vi "PID_Trajectory tracking_0125.vi"() -> ()   [LabVIEW 2018]
doc: "Demonstrates the use of the Network Streams functions to send LED status to the myRIO target."
uses:
  <vilib>/ErrorRing/Error Ring.xnode
  <vilib>/vision/NI_Vision_Development_Module.lvlib
panel:
  out "e(t-1)":dbl[](array[numeric])
  out "Ki part":dbl[](array[numeric])
  out "Kd part":dbl[](array[numeric])
  out "Kp part":dbl[](array[numeric])
  out "desired_relative_end_point_y":dbl
  out "desired_relative_end_point_x":dbl
  out "predicted_output_pr":dbl
  out "predicted_output_dr":dbl
  out "u(t)":dbl[](array[numeric])
  in  "Ki: Intergrate":dbl
  in  "Kd: Derivative":dbl[](array[numeric])
  in  "T":dbl[](array[numeric])
  in  "Kp: Proportional":dbl[](array[numeric])
  out "error  e(t)":dbl[](array[numeric])
  out "error_end_point_y":dbl
  out "error_end_point_x":dbl
  out "relative_end_point_y":dbl
  out "relative_end_point_x":dbl
  out "magnet_input_pr":dbl
  out "magnet_input_dr":dbl
  in  "打开仅尖端轨迹":bool
  out "仅尖端轨迹":T1(plugin-control)
  out "Bounding Box.Y Top":i32
  out "Bounding Box.X Left":i32
  out "curve_min_y":dbl
  out "curve_min_x":dbl
  out "curve_max_y":dbl
  out "curve_max_x":dbl
  out "relative_end_point_y":dbl
  out "relative_end_point_x":dbl
  out "delta_y":dbl
  out "delta_x":dbl
  out "pr":dbl
  out "tan(v)":dbl
  out "delta_velocity":dbl format="%#_10g"
  out "delta_time":dbl
  out "now time":timestamp[](array[timestamp])
  out "prev time":timestamp[](array[timestamp])
  out "delta_distance":dbl
  out "prev_end_point_y":dbl
  out "prev_end_point_x":dbl
  out "now_end_point_y":dbl
  out "now_end_point_x":dbl
  out "prev_end_point_y":dbl[](array[numeric])
  out "prev_end_point_x":dbl[](array[numeric])
  out "dr":dbl
  in  "Ar":sgl=11.0
  out "all parameters":dbl[][](array[numeric])
  out "direction angle":sgl[](array[numeric])
  out "dr":sgl
  out "strength":dbl[](array[numeric])
  out "场强":dbl
  out "end_point_y":T2
  out "end_point_x":dbl[](array[numeric])
  out "start_point_y":dbl[](array[numeric])
  out "start_point_x":dbl[](array[numeric])
  out "T":i32[](array[numeric])
  out "c":dbl[](array[numeric])
  out "b":dbl[](array[numeric])
  out "a\na":dbl[](array[numeric])
  out "c":dbl
  out "b":dbl
  out "a":dbl
  out "Angles (deg)":sgl[](array[numeric]) format="%.2f"
  in  "wr":sgl
  in  "打开轨迹":bool
  out "中心轨迹和尖端轨迹":T1(plugin-control)
  out "end_y":dbl
  out "end_x":dbl
  out "start_y":dbl
  out "start_x":dbl
  out "Image Pixels (U8)":u8[][](array[numeric])
  in  "Poly":dbl
  out "中心轨迹":T1(plugin-control)
  in  "保存按钮":bool
  out "Object Center":cluster{"X":sgl, "Y":sgl}
  out "黑白图":T1(plugin-control)
  in  "Number of Erosion":i32=5
  in  "Settings":T3={"Objects"=1, "Threshold"=128, "Reject Border"=FALSE, "Fill Holes"=FALSE, "Min Object Size"=TRUE, "Min Size"=5500, "Max Object Size"=FALSE, "Max Size"=100, "Show Search Area"=TRUE, "Show Center"=TRUE, "Show Bounding Box"=TRUE} {"Objects" items=["Bright Objects", "Dark Objects"]; "Threshold" min=1 max=999999999 step=1; "Max Size" min=1 max=999999999 step=1; "Min Size" min=1 max=999999999 step=1}
  out "Objects":T4(array[cluster]) {"Aspect Ratio" format="%.2f"; "Orientation" format="%.2f"; "Area" format="%.2f"; "Object Center"."Y" format="%.2f"; "Object Center"."X" format="%.2f"}
  in  "Search Rect (entire image)":T5={"Left"=160, "Top"=740, "Right"=1900, "Bottom"=1620, "Rotation"=0.0} {"Rotation" format="%.2f"; "Left" scale=0.0..1024.0; "Right" scale=0.0..1024.0}
  in  "Range":cluster{"Lower value":sgl, "Upper value":sgl}={"Lower value"=170.0, "Upper value"=255.0} {"Upper value" format="%.2f"; "Lower value" format="%.2f"}
  out "原图":T1(plugin-control)
  in  "停止":bool
  out "T":i32
  out "T":i32
  in  "磁场变换":bool=TRUE
  in  "Pause":bool
  out "Array":dbl[](array[numeric])
  in  "Parameter Settings":T6(tab)=enum."Rotating Field" caption="Field Types"
  in  "Ag":dbl
  in  "dg":dbl
  in  "pg":dbl
  in  "fg":dbl
  in  "AoOF":dbl
  in  "fo":sgl
  in  "do":sgl
  in  "oo":sgl
  in  "po":sgl
  in  "cc":sgl
  in  "pc":sgl
  in  "wc":sgl
  in  "dc":sgl
  in  "Ac":dbl
  in  "Dis phase step":dbl
  in  "Dis phase frequency (Hz)":dbl
  in  "Dis tumbling frequency (Hz)":dbl
  in  "Dis strength(mT)":dbl
  in  "Swa strength (mT)":dbl
  in  "Swa frequency (Hz)":dbl
  in  "Swa pitch angle (deg)":dbl
  in  "Swa direction angle (deg)":dbl
  in  "Swa ratio":dbl=1.0
  in  "Pitch Angle (rotating around Constant, deg)":dbl
  in  "Ratio (A/C)":sgl
  in  "Direction Angle (deg)":sgl
  in  "Pitch Angle (rotating around Origin, deg)":sgl
  in  "Frequency (Hz)":sgl
  in  "Strength (mT)":dbl
  in  "Ar 2":dbl caption="Ar"
  in  "ratio":sgl
  in  "pr  2":sgl
  in  "dr  2":sgl
  in  "wr  2":sgl
  in  "p_x":sgl
  out "Numeric 5":i32
  in  "Stop":bool
  out "error out":errorcluster
  in  "Target IP Address":string="172.22.11.2"
  # "Overview: Magnetic field calculation, and send parameters to myRIO\nInstructions:\n1. Verify the value of Target IP Address. Set Visa resource name.\n2. Ensure RT Main.vi is already running. \n3. Run this VI. Set parameters of magnetic field."
  # "Strength (mT)"
  # "Frequency (Hz)"
  # "Pitch Angle (deg)"
  # "Direction Angle (deg)"
  # "Strength (mT)"
  # "Pitch Angle (deg)"
  # "Direction Angle (deg)"
  # "Frequency (Hz)"
  # "Strength (mT)"
  # "Oscilation Frequency (Hz)"
  # "Oscilation Angle (deg)"
  # "Pitch Angle (deg)"
  # "Direction Angle (deg)"
  # "Strength (mT)"
  # "Frequency (Hz)"
  # "Pitch Angle (deg)"
  # "Direction Angle (deg)"
  # "Conical Angle (deg)"
  # "Strength (mT)"
  # "Tumbling Frequency (Hz)"
  # "Phase Frequency (Hz)"
  # "Phase Step"
  # "Strength (mT)"
  # "Frequency (Hz)"
  # "Pitch Angle (deg)"
  # "Direction Angle (deg)"
  # "Ratio"
  # "Strength (mT)"
  # "Frequency (Hz)"
  # "Ratio (A/C)"
  # "Direction Angle (deg)"
  # "Pitch Angle (rotating around Origin, deg)"
  # "Pitch Angle (rotating around Constant, deg)"
  # "Strength (mT)"
  # "Frequency (Hz)"
  # "Pitch Angle Y (deg)"
  # "Pitch Angle X (deg)"
  # "Direction Angle (deg)"
  # "ratio (l/s)"
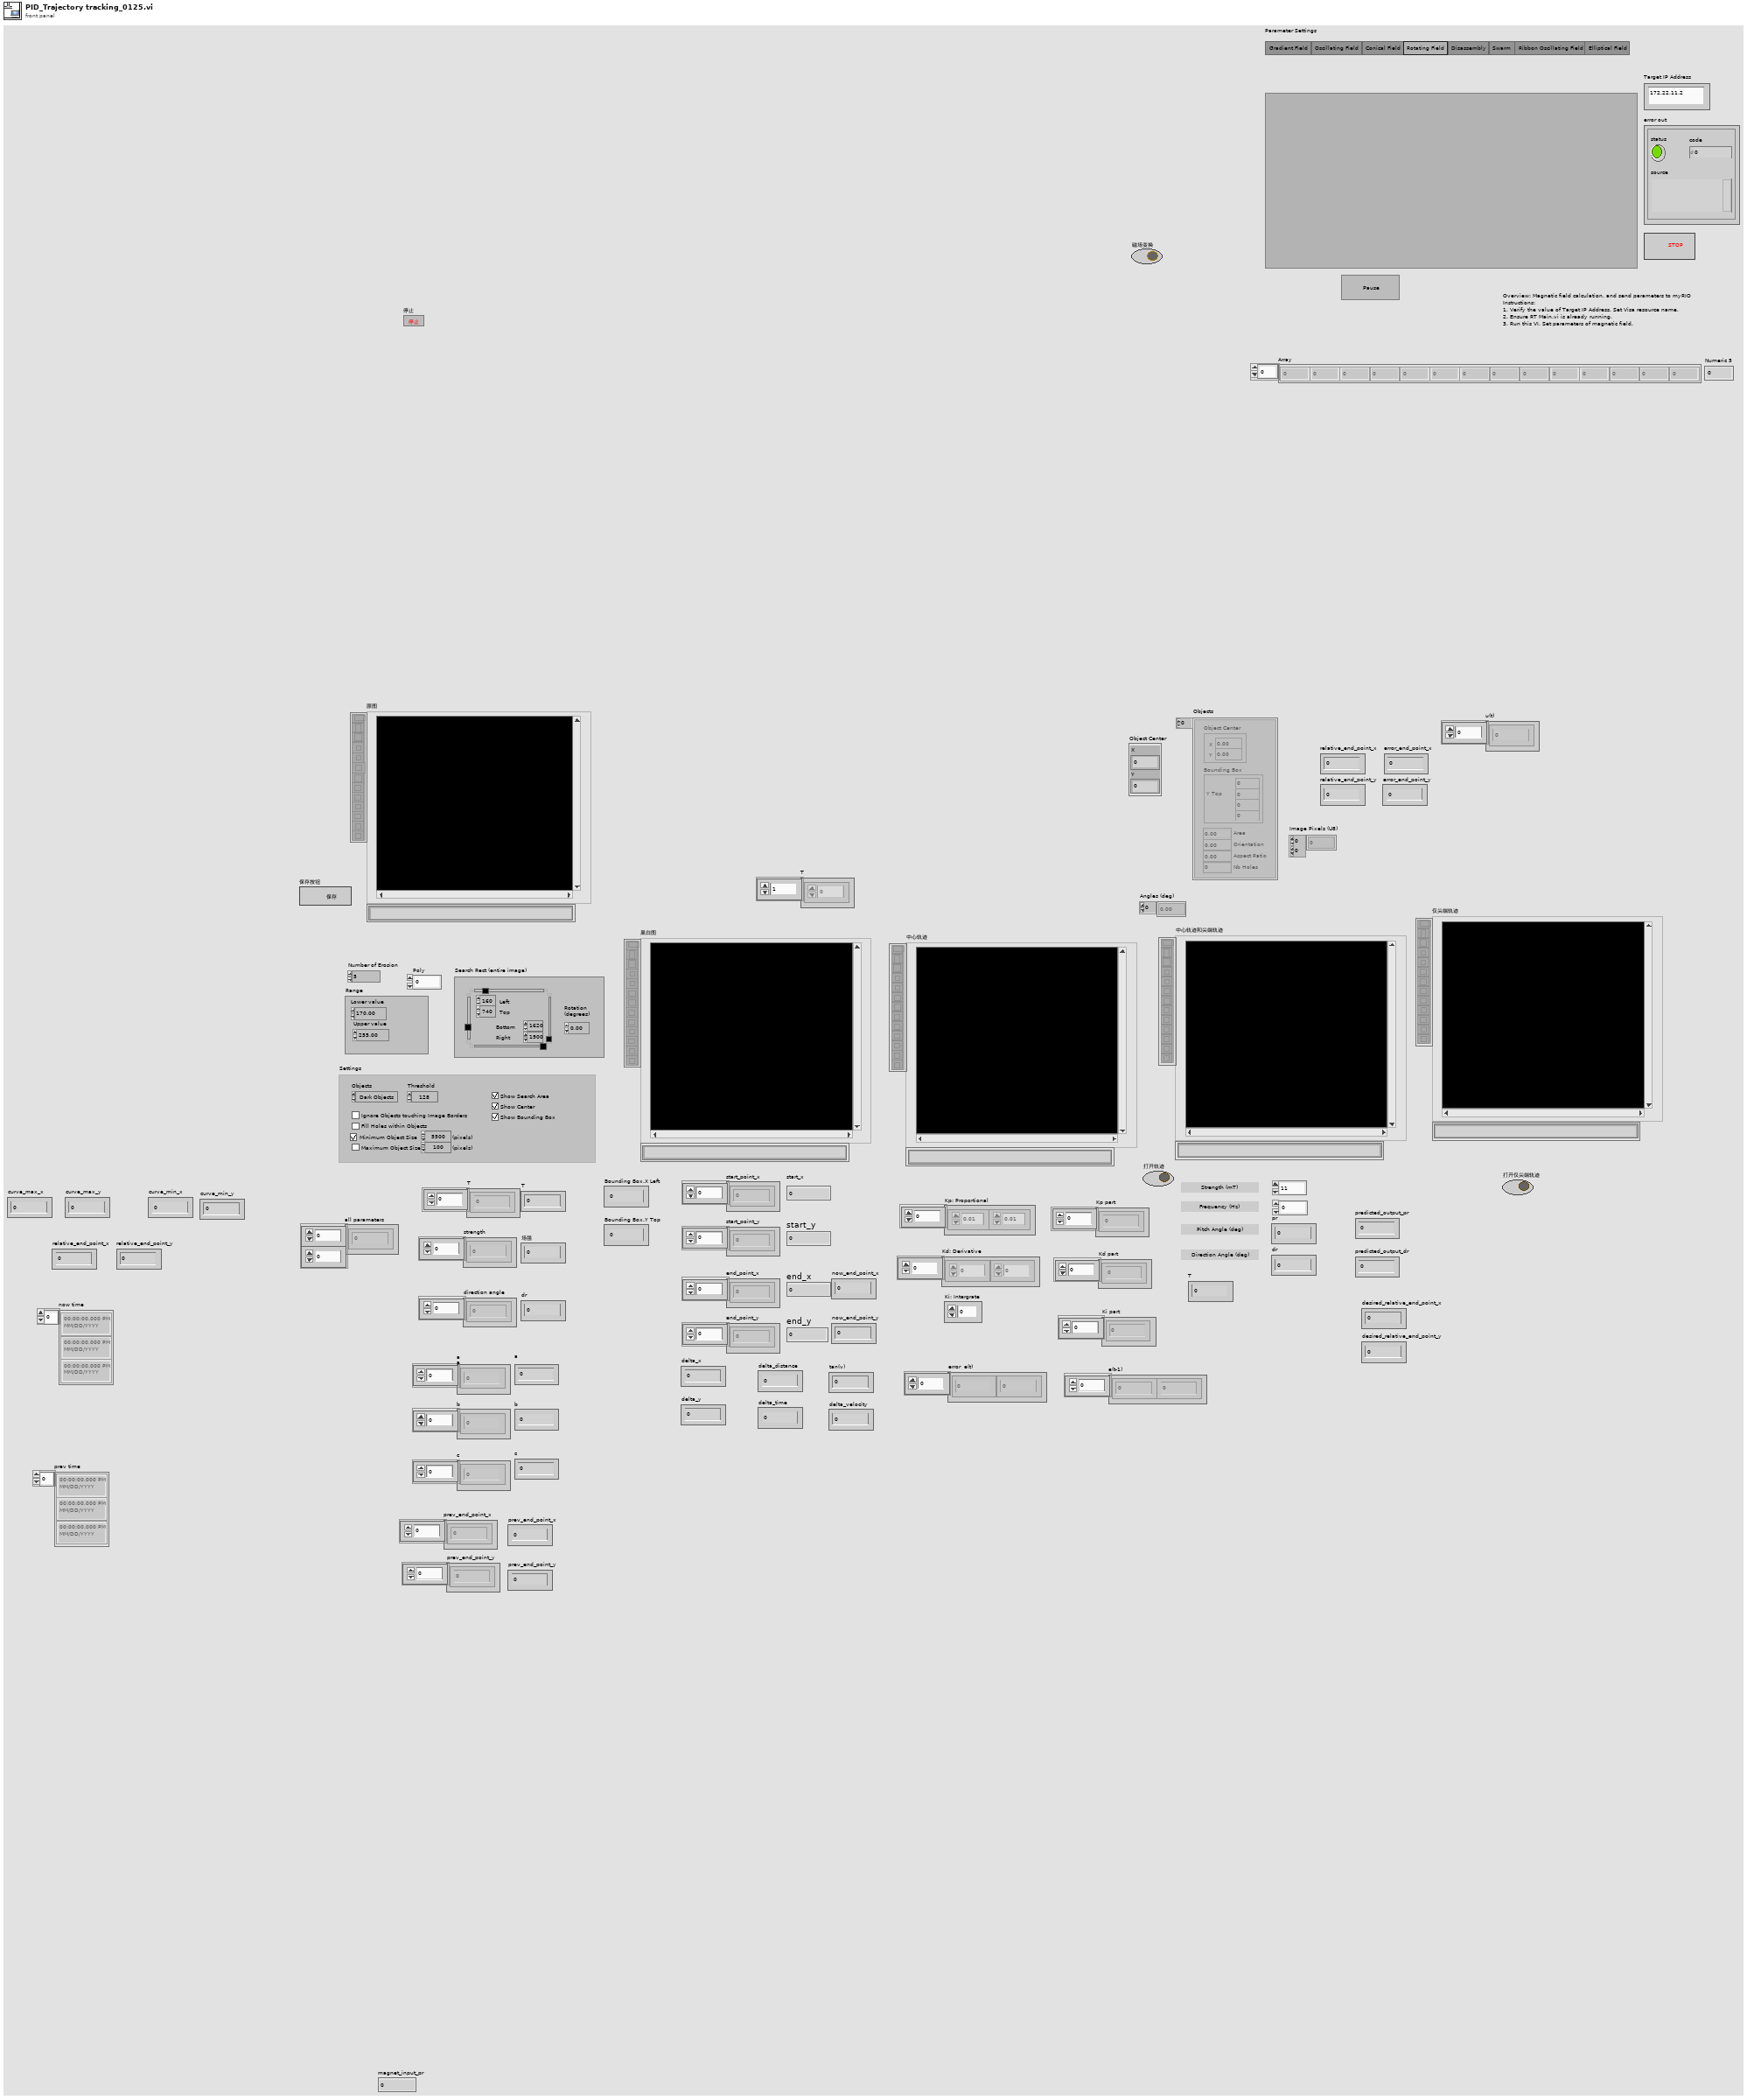
[diagram p1: front panel]
types:
  T1 = typedef "IMAQ Image.ctl" = refnum<image>
  T2 = typedef "控件 3.ctl" = dbl[]
  T3 = cluster{"Objects":u16, "Threshold":i32, "Reject Border":bool, "Fill Holes":bool, "Min Object Size":bool, "Min Size":i32, "Max Object Size":bool, "Max Size":i32, "Show Search Area":bool, "Show Center":bool, "Show Bounding Box":bool}
  T4 = cluster{"Object Center":cluster{"X":sgl, "Y":sgl}, "Bounding Box":cluster{"X Left":i32, "Y Top":i32, "X Right":i32, "Y Bottom":i32}, "Area":sgl, "Orientation":sgl, "Aspect Ratio":sgl, "Nb Holes":i32}[]
  T5 = typedef "IMAQ Rectangle" = cluster{"Left":i32, "Top":i32, "Right":i32, "Bottom":i32, "Rotation":dbl}
  T6 = enum32{"Gradient Field ", "Oscillating Field", "Conical Field", "Rotating Field", "Disassembly", "Swarm", "Ribbon Oscillating Field", "Elliptical Field"}
  T7 = typedef "Image Type" = u32
  T8 = cluster{"Object Center":cluster{"X":sgl, "Y":sgl}, "Bounding Box":cluster{"X Left":i32, "Y Top":i32, "X Right":i32, "Y Bottom":i32}, "Area":sgl, "Orientation":sgl, "Aspect Ratio":sgl, "Nb Holes":i32}
  T9 = cluster{"X Left":i32, "Y Top":i32, "X Right":i32, "Y Bottom":i32, "Rotation":dbl}
  T10 = typedef "ROI Descriptor" = cluster{"Global Rectangle":i32[], "Contours":cluster{"ID":enum32{"External", "Internal"}, "Type":u32, "Coordinates":i32[]}[]}
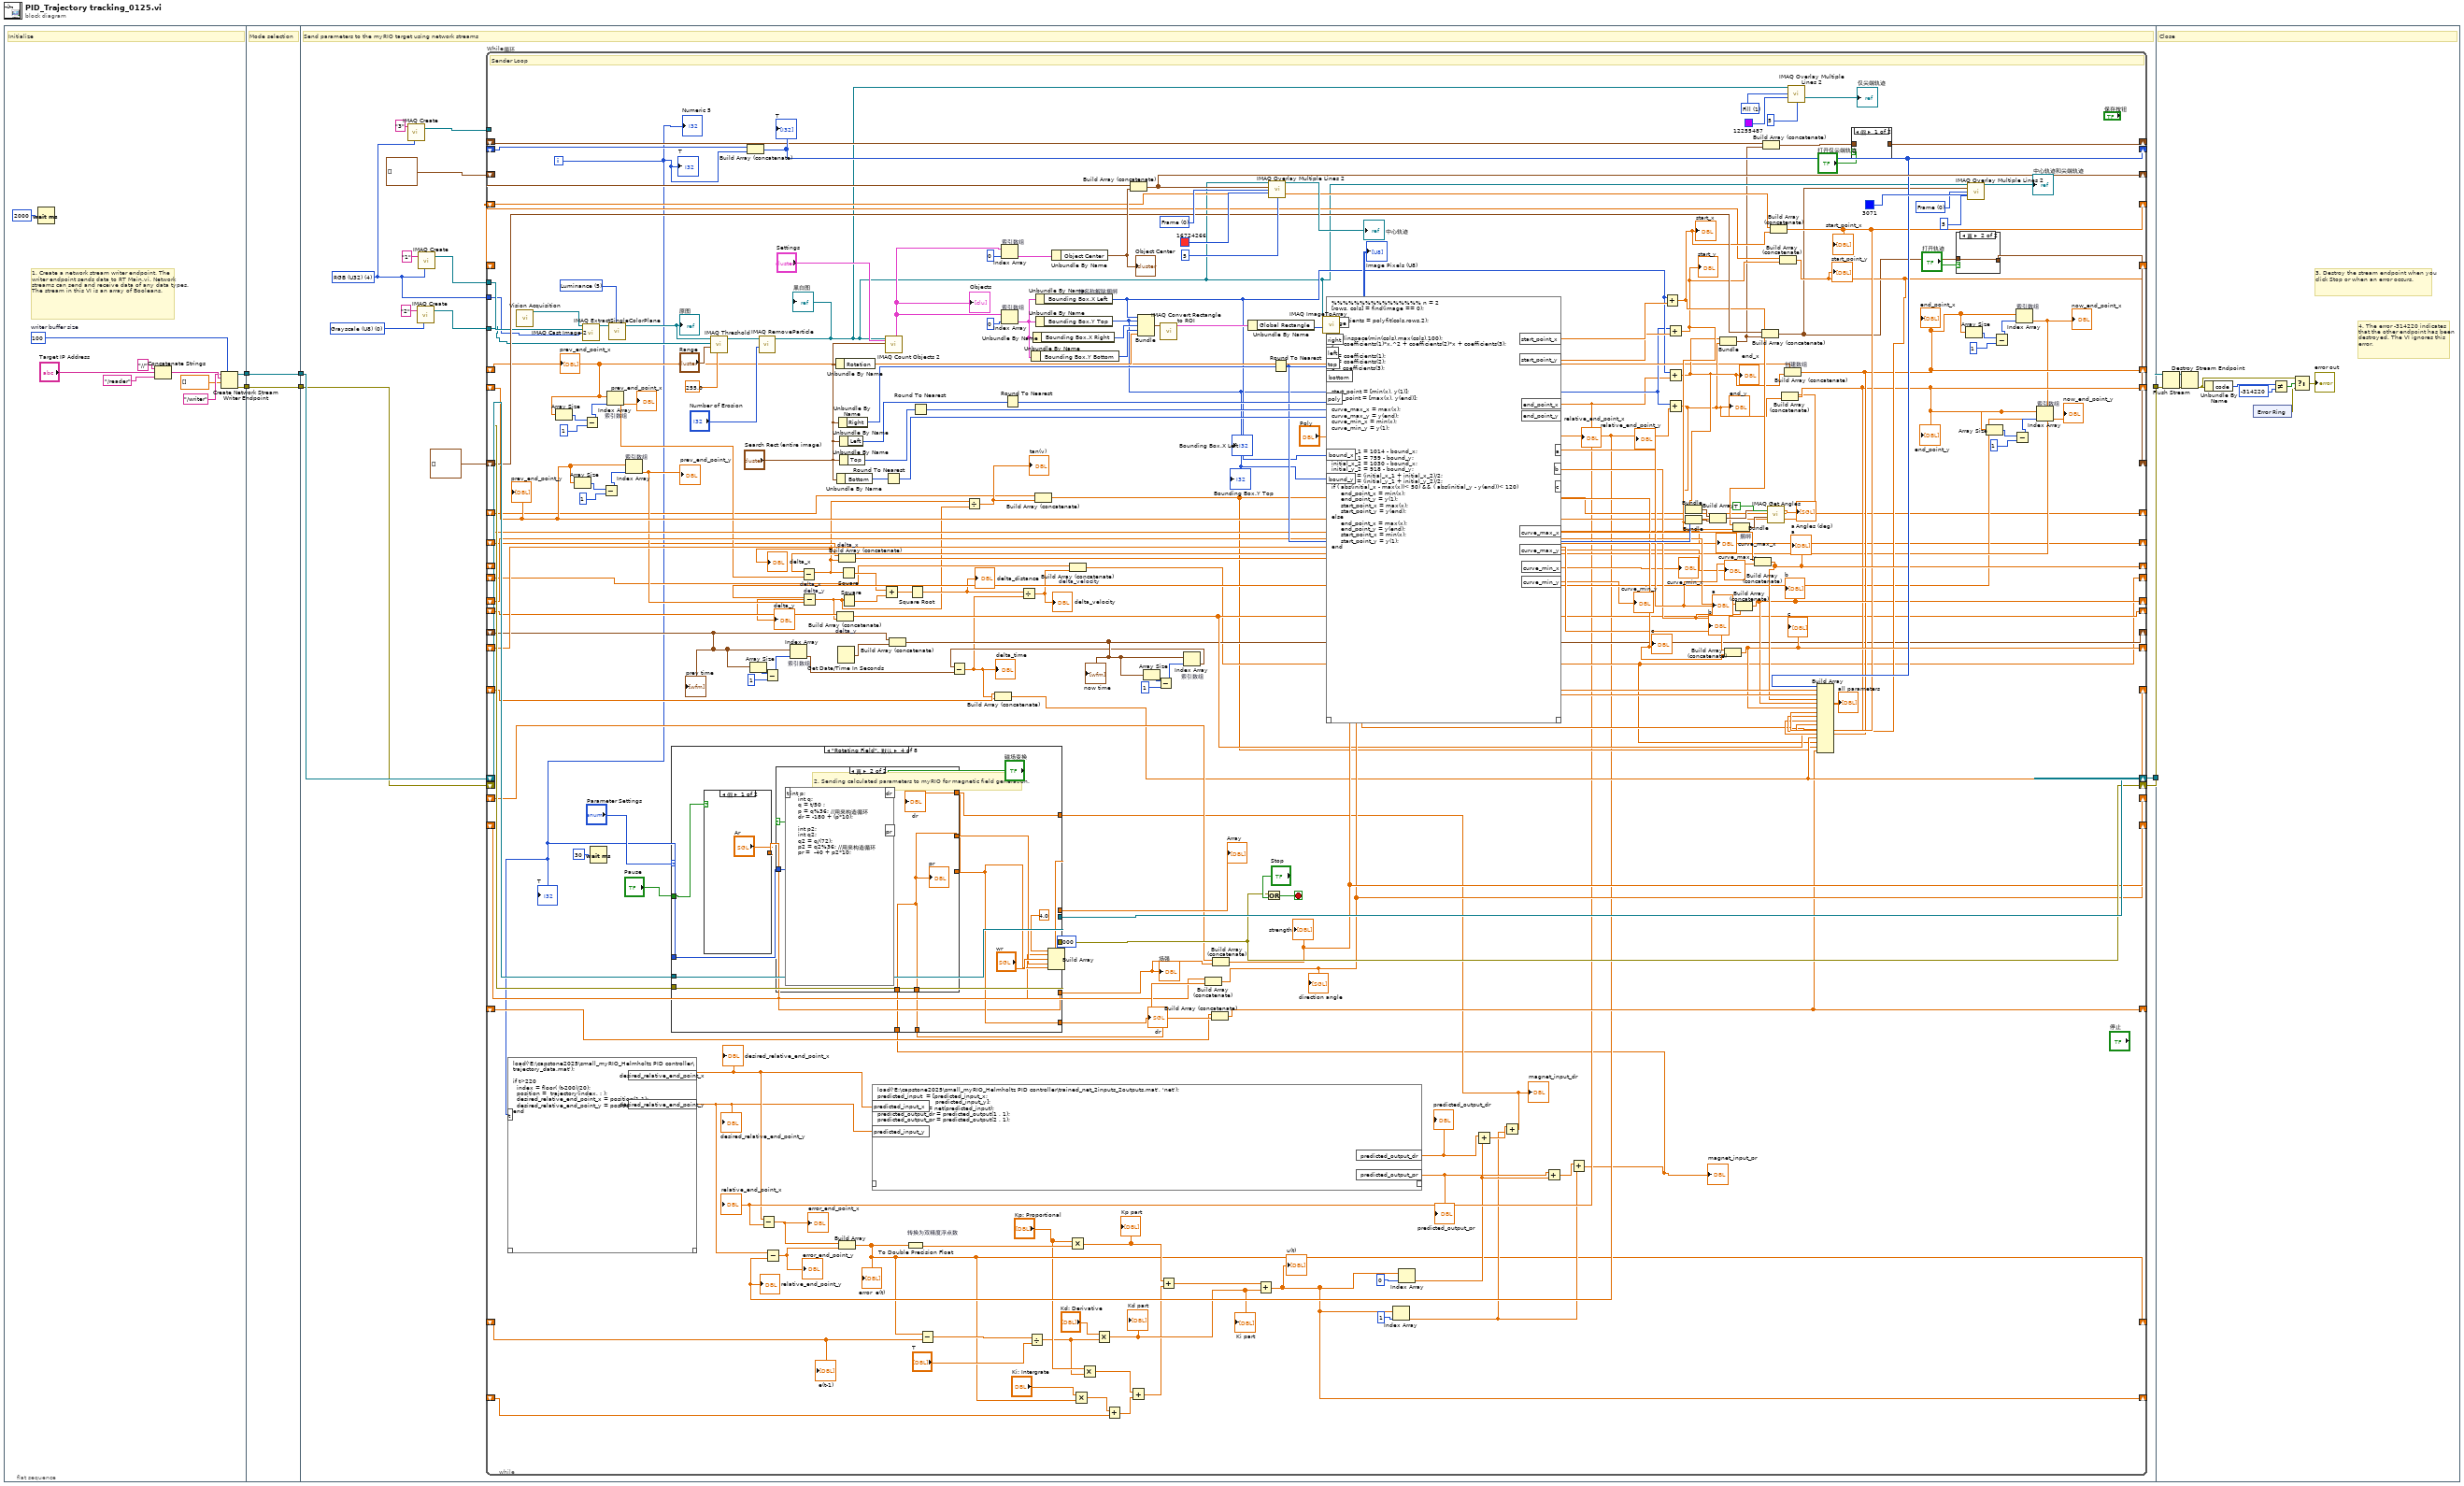
[diagram p0: block diagram]
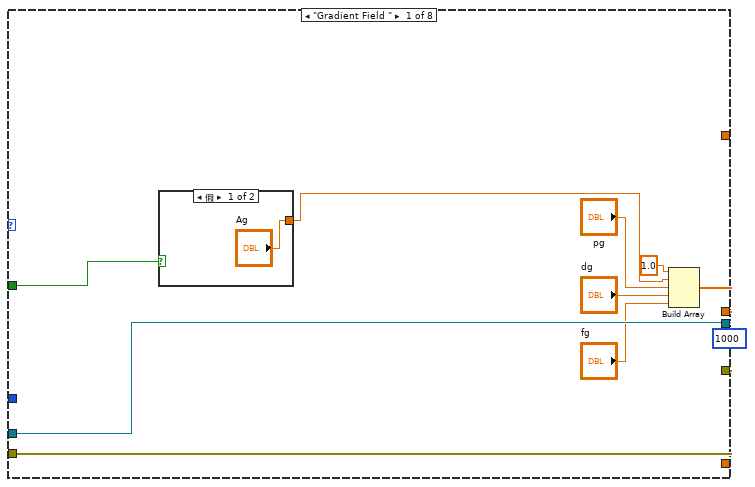
[diagram p4: hidden frame]
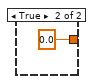
[diagram p5: hidden frame]
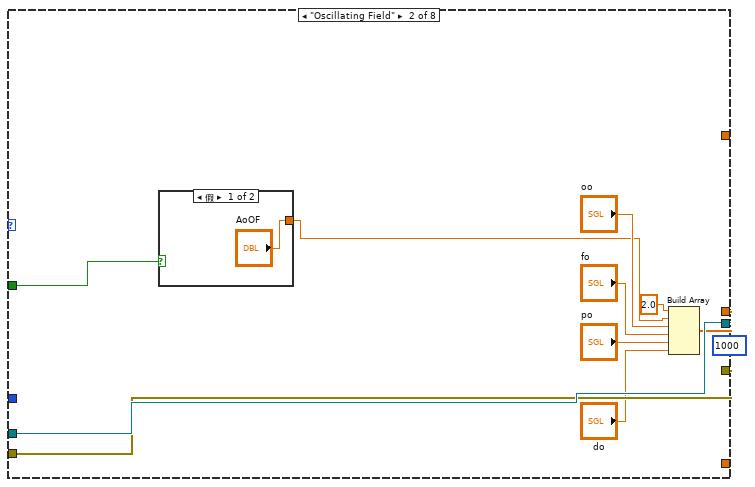
[diagram p6: hidden frame]
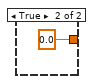
[diagram p7: hidden frame]
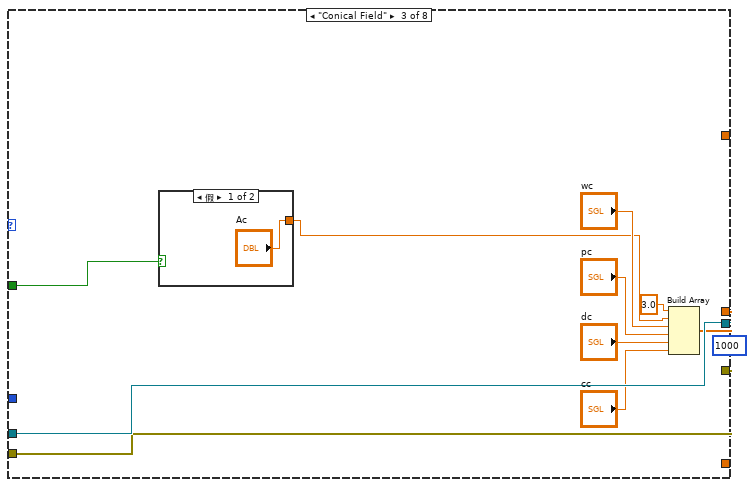
[diagram p8: hidden frame]
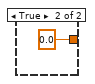
[diagram p9: hidden frame]
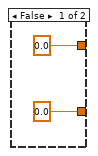
[diagram p10: hidden frame]
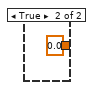
[diagram p11: hidden frame]
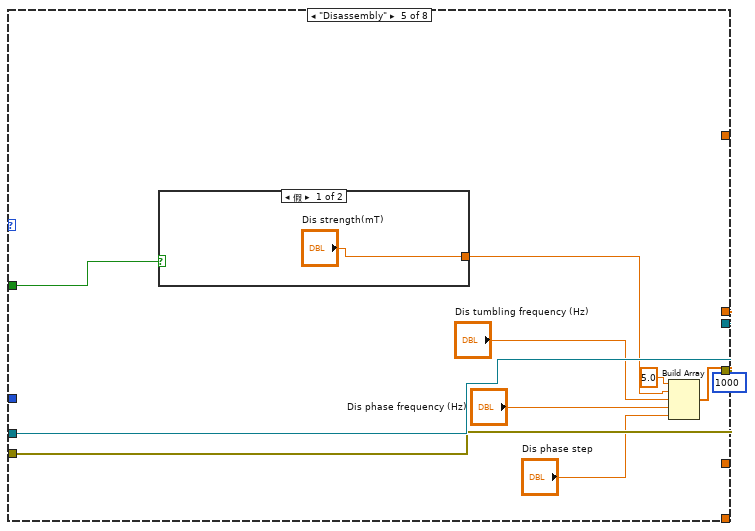
[diagram p12: hidden frame]
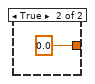
[diagram p13: hidden frame]
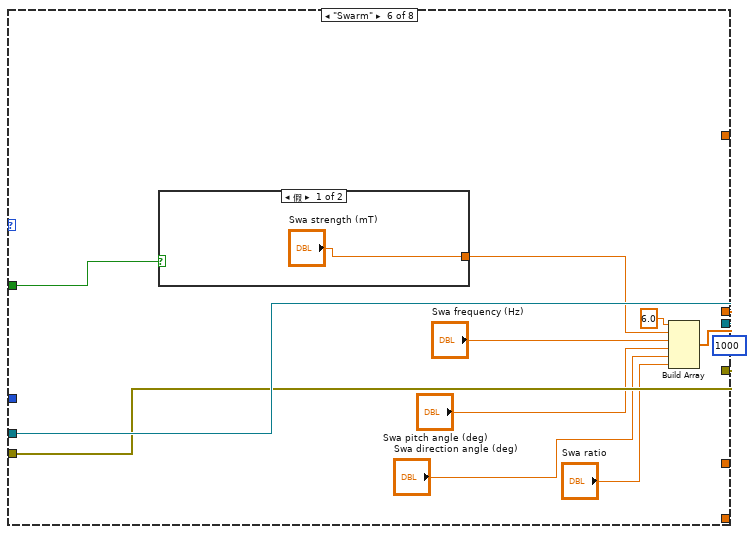
[diagram p14: hidden frame]
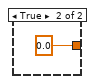
[diagram p15: hidden frame]
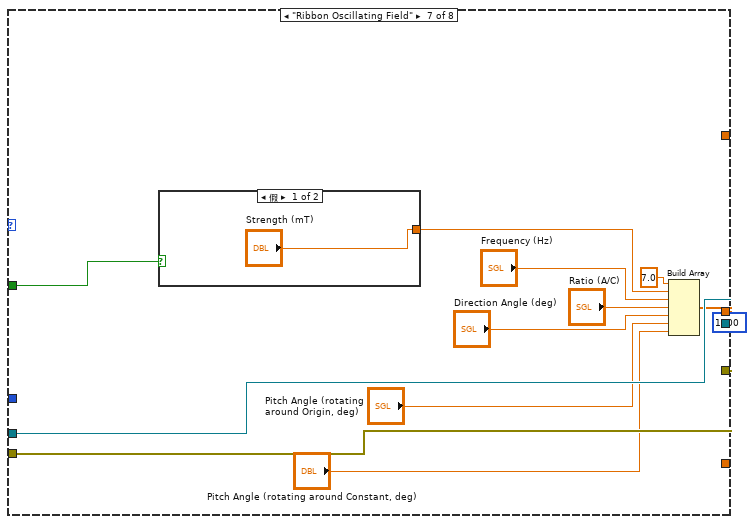
[diagram p16: hidden frame]
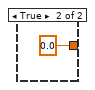
[diagram p17: hidden frame]
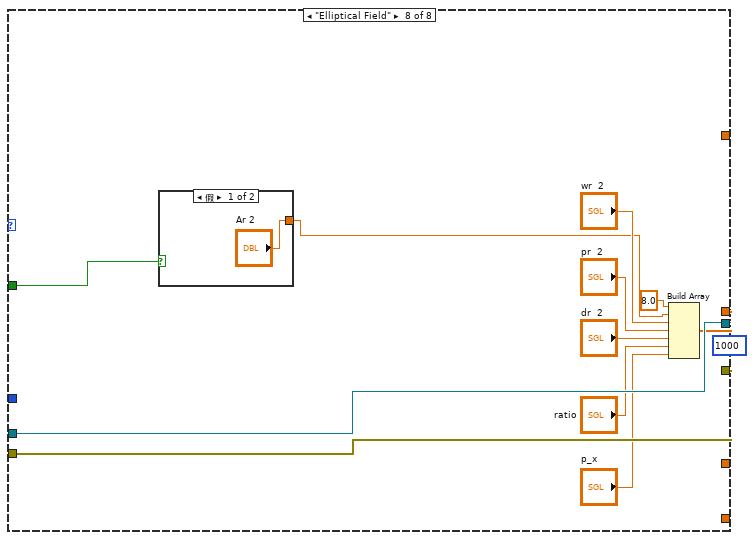
[diagram p18: hidden frame]
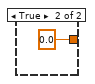
[diagram p19: hidden frame]
diagram:
  n1 = flat-sequence {
    tunnel: [w11] -> w2
    tunnel: [w10] -> w1
    tunnel: [w18] -> w4
    tunnel: [w17] -> w3
    tunnel: w1 -> [w17]
    tunnel: w2 -> [w18]
    tunnel: [w30] -> w6
    tunnel: w4 -> [w32]
    tunnel: [w29] -> w5
    tunnel: w3 -> [w31]
    tunnel: w6 -> [w370]
    tunnel: w5 -> [w367]
    frame #0 {
      w9 = 100  # writer buffer size
      # "1. Create a network stream writer endpoint. The writer endpoint sends data to RT Main.vi. Network streams can send and receive data of any data types. The stream in this VI is an array of Booleans."
      # "Initialize"
      n2 = Wait (ms)(milliseconds to wait=2000) -> ()  [unwired: 1 out]
      n3 = Concatenate Strings("//", "Target IP Address", "/reader") -> (w16:string)
      n4 = Create Network Stream Writer Endpoint(7:w9, 9:dbl[] [], 10:w16, 11:"/writer" ("reader name")) -> (0:w10:errorcluster, 3:w11:refnum<k21>)  [unwired: 3 in]
    }
    frame #1 {
      # "Mode selection"
    }
    frame #2 {
      w26 = T7 0 items=["Grayscale (U8)", "Grayscale (I16)", "Grayscale (SGL)", "Complex (CSG)", "RGB (U32)", "HSL (U32)", "RGB (U64)", "Grayscale (U16)"] ("Image Type")
      w19 = T7 4 items=["Grayscale (U8)", "Grayscale (I16)", "Grayscale (SGL)", "Complex (CSG)", "RGB (U32)", "HSL (U32)", "RGB (U64)", "Grayscale (U16)"] ("Image Type")
      # "Send parameters to the myRIO target using network streams"
      n5 = call "IMAQ Create"("Image Name"="3", "Image Type"=w19) -> ("New Image"=w22:T1)  [unwired: 3 in, 1 out]
      n6 = call "IMAQ Create"("Image Name"="2", "Image Type"=w26) -> ("New Image"=w24:T1)  [unwired: 3 in, 1 out]
      n7 = call "IMAQ Create"("Image Name"="1", "Image Type"=w19) -> ("New Image"=w25:T1)  [unwired: 3 in, 1 out]
      n8 = while "While循环" {
        shift-right: [w225] -> w29
        shift-left: w31 -> [w227]
        shift-right: [w226] -> w30
        shift-left: w32 -> [w228]
        tunnel: w25 -> [w176]
        tunnel: w24 -> [w175]
        tunnel: w22 -> [_]
        shift-right: [w172] -> _
        shift-left: cluster{"X":dbl, "Y":dbl}[] [] -> [w177]
        shift-right: [w178] -> _
        shift-left: cluster{"X":dbl, "Y":dbl}[] [] -> [w179]
        tunnel: w19 -> [w174]
        shift-right: [w144] -> _
        shift-left: _ -> [w164]
        shift-right: [w139] -> _
        shift-left: _ -> [w162]
        shift-right: [w143] -> _
        shift-left: _ -> [w159]
        shift-right: [w147] -> _
        shift-left: _ -> [w158]
        shift-right: [w142] -> _
        shift-left: _ -> [w156]
        shift-right: [w141] -> _
        shift-left: _ -> [w154]
        shift-right: [w135] -> _
        shift-left: _ -> [w127]
        shift-right: [w131] -> _
        shift-left: _ -> [w123]
        shift-right: [w146] -> _
        shift-left: _ -> [w150]
        shift-right: [w145] -> _
        shift-left: _ -> [w148]
        shift-right: [w112] -> _
        shift-left: _ -> [w114]
        shift-right: [w111] -> _
        shift-left: _ -> [w113]
        shift-right: [w101] -> _
        shift-left: _ -> [w106]
        shift-right: [w98] -> _
        shift-left: _ -> [w99]
        shift-right: [w94] -> _
        shift-left: _ -> [w95]
        shift-right: [w89] -> _
        shift-left: _ -> [w90]
        shift-right: [w79] -> _
        shift-left: _ -> [w80]
        shift-right: [w73] -> _
        shift-left: _ -> [w74]
        shift-right: [w41] -> _
        shift-left: _ -> [w62]
        shift-right: [w45] -> _
        shift-left: _ -> [w44]
        i -> [w54]
        stop <- w221 stop-if-true
        w75 = u32 1 items=["Frame", "Fill"] ("Drawing Mode (Frame)")
        w82 = u32 0 items=["Frame", "Fill"] ("Drawing Mode (Frame)")
        w208 = u32 0 items=["Frame", "Fill"] ("Drawing Mode (Frame)")
        w218 = 5 items=["Red", "Green", "Blue", "Hue", "Saturation", "Luminance", "Value", "Intensity"] ("Color Plane")
        # "2. Sending calculated parameters to myRIO for magnetic field generation."
        # "Sender Loop"
        n9 = script code="load('E:\\capstone2025\\small_myRIO_Helmholtz PID controller\\trajectory_data.mat');\n\nif t>220\n  index = floor( (t-200)/20);\n  position =  trajectory(index, : );\n  desired_relative_end_point_x = position(1,1);\n  desired_relative_end_point_y = position(1,2);\nend"("t"=w54) -> ("desired_relative_end_point_x"=w35:dbl, "desired_relative_end_point_y"=w34:dbl)  [unwired: 1 in, 1 out]
        "desired_relative_end_point_x" <- w35
        "desired_relative_end_point_y" <- w34
        n10 = call "Vision Acquisition"() -> ("Image Out"=w206:T1)  [unwired: 23 in, 4 out]
        n11 = Array Size(array=w127) -> (size(s)=w129:i32)
        n12 = Array Size(array=w123) -> (size(s)=w125:i32)
        n13 = call "IMAQ Cast Image 2"("Image Src"=w206, "Image Dst"=w176, "Image Type"=w174) -> ("Image Dst Out"=w219:T1)  [unwired: 11 in, 1 out]
        n14 = Subtract(x=w129, y=1) -> (x-y=w128:i32)
        n15 = Wait (ms)(milliseconds to wait=u32 30 ("等待时间（毫秒）")) -> ()  [unwired: 1 out]
        n16 = Subtract(x=w125, y=1) -> (x-y=w124:i32)
        n17 = Index Array "索引数组"(array=w127, index=w128) -> (element=w121:dbl)
        "prev_end_point_x" <- w121
        n18 = call "IMAQ ExtractSingleColorPlane"("Color Plane"=w218, "Image Src"=w219) -> ("Image Dst Out"=w217:T1)  [unwired: 8 in, 1 out]
        "原图" <- w217
        n19 = Index Array "索引数组"(array=w123, index=w124) -> (element=w120:dbl)
        "prev_end_point_y" <- w120
        n20 = call "IMAQ Threshold"("Replace Value"=sgl 255.0, "Range"="Range", "Image Dst"=w175, "Image Src"=w217) -> ("Image Dst Out"=w205:T1)  [unwired: 6 in, 1 out]
        n21 = Build Array (concatenate)(w158, w54) -> (w147:i32[])
        "T" <- w147
        n22 = Array Size(array=w106) -> (size(s)=w109:i32)
        n23 = call "IMAQ RemoveParticle"("Number of Erosion"="Number of Erosion", "Image Src"=w205) -> ("Image Dst Out"=w71:T1)  [unwired: 8 in, 1 out]
        "黑白图" <- w71
        n24 = Subtract(x=w109, y=1) -> (x-y=w108:i32)
        n25 = Index Array "索引数组"(array=w106, index=w108) -> (element=w105:timestamp)
        n26 = Unbundle By Name("Search Rect (entire image)") -> ("Rotation"=w202:dbl)
        n27 = Unbundle By Name("Search Rect (entire image)") -> ("Bottom"=w186:i32)
        n28 = Get Date/Time In Seconds() -> (seconds since 1Jan1904=w110:timestamp)
        n29 = Unbundle By Name("Search Rect (entire image)") -> ("Right"=w190:i32)
        n30 = Unbundle By Name("Search Rect (entire image)") -> ("Left"=w189:i32)
        n31 = Unbundle By Name("Search Rect (entire image)") -> ("Top"=w188:i32)
        n32 = script code="load('E:\\capstone2025\\small_myRIO_Helmholtz PID controller\\trained_net_2inputs_2outputs.mat', 'net');\npredicted_input  = [predicted_input_x; \n                               predicted_input_y];\npredicted_output = net(predicted_input);\npredicted_output_dr = predicted_output(1 , 1);\npredicted_output_pr = predicted_output(2 , 1);"("predicted_input_y"=w34, "predicted_input_x"=w35) -> ("predicted_output_dr"=w53:dbl, "predicted_output_pr"=w50:dbl)  [unwired: 1 in, 1 out]
        "predicted_output_dr" <- w53
        "predicted_output_pr" <- w50
        n33 = Round To Nearest(number=w186) -> (nearest integer value=w185:i32)
        n34 = call "IMAQ Count Objects 2"("Settings"="Settings", "Search Rect (entire image)"="Search Rect (entire image)", "Image"=w71) -> ("Objects"=w204:T4)  [unwired: 4 in, 4 out]
        "Objects" <- w204
        n35 = Build Array (concatenate)(w106, w110) -> (w101:timestamp[])
        "now time" <- w101
        n36 = Round To Nearest(number=w188) -> (nearest integer value=w187:i32)
        n37 = Index Array "索引数组"(array=w204, index=0 ("索引")) -> (element=w211:T8)
        n38 = Index Array "索引数组"(array=w204, index=0 ("索引")) -> (element=w200:T8)
        n39 = Round To Nearest(number=w189) -> (nearest integer value=w182:i32)
        n40 = Unbundle By Name(w200) -> ("Bounding Box.Y Bottom"=w194:i32)
        n41 = Unbundle By Name(w200) -> ("Bounding Box.X Right"=w195:i32)
        n42 = Unbundle By Name "按名称解除捆绑"(w200) -> ("Bounding Box.X Left"=w84:i32)
        "Bounding Box.X Left" <- w84
        n43 = Unbundle By Name(w200) -> ("Bounding Box.Y Top"=w83:i32)
        "Bounding Box.Y Top" <- w83
        n44 = Unbundle By Name(w211) -> ("Object Center"=w210:cluster{"X":sgl, "Y":sgl})
        "Object Center" <- w210
        n45 = Build Array (concatenate)(w179, w210) -> (w178:cluster{"X":dbl, "Y":dbl}[])
        n46 = Bundle("X Left"=w84, "Y Top"=w83, "X Right"=w195, "Y Bottom"=w194, "Rotation"=w202) -> (w201:T9)  [unwired: 1 in]
        n47 = Array Size(array=w101) -> (size(s)=w104:i32)
        n48 = Subtract(x=w104, y=1) -> (x-y=w103:i32)
        n49 = call "IMAQ Convert Rectangle to ROI"("Rectangle"=w201) -> ("ROI Descriptor"=w199:T10)  [unwired: 8 in, 1 out]
        n50 = Index Array "索引数组"(array=w101, index=w103) -> (element=w100:timestamp)
        n51 = Subtract(x=w100, y=w105) -> (x-y=w97:dbl)
        "delta_time" <- w97
        n52 = Build Array (concatenate)(w99, w97) -> (w98:dbl[])
        n53 = Unbundle By Name(w199) -> ("Global Rectangle"=w184:i32[])
        n54 = call "IMAQ Overlay Multiple Lines 2"("Image"=w71, "Line End Points"=w178, "Drawing Mode (Frame)"=w208, "Color"=u32 16724266, "Width"=u32 5) -> ("Image Out"=→"中心轨迹":T1)  [unwired: 9 in, 1 out]
        n55 = Round To Nearest(number=w190) -> (nearest integer value=w165:i32)
        n56 = call "IMAQ ImageToArray"("Optional Rectangle"=w184, "Image"=w71) -> ("Image Pixels (U8)"=w196:u8[][])  [unwired: 2 in, 4 out]
        "Image Pixels (U8)" <- w196
        n57 = script code="%%%%%%%%%%%%%%%% n = 2\n[rows, cols] = find(image == 0);\n\ncoefficients = polyfit(cols,rows,2);\n\n\nx = linspace(min(cols),max(cols),100); \ny = coefficients(1)*x.^2 + coefficients(2)*x + coefficients(3);\n\na = coefficients(1);\nb = coefficients(2);\nc = coefficients(3);\n\n\n\nstart_point = [min(x), y(1)];  \nend_point = [max(x), y(end)];\n\ncurve_max_x = max(x);\ncurve_max_y = y(end);\ncurve_min_x = min(x);\ncurve_min_y = y(1);\n\n\n\ninitial_x_1 = 1014 - bound_x; \ninitial_y_1 = 759 - bound_y;\ninitial_x_2 = 1030 - bound_x;\ninitial_y_2 = 918 - bound_y;\ninitial_x = (initial_x_1 + initial_x_2)/2;\ninitial_y = (initial_y_1 + initial_y_2)/2;\nif ( abs(initial_x - max(x))< 50) && ( abs(initial_y - y(end))< 120)\n     end_point_x = min(x);\n     end_point_y = y(1);\n     start_point_x = max(x);\n     start_point_y = y(end);\nelse\n     end_point_x = max(x);\n     end_point_y = y(end);\n     start_point_x = min(x);\n     start_point_y = y(1);\nend"("image"=w196, "poly"="Poly", "right"=w165, "left"=w182, "top"=w187, "bottom"=w185, "bound_x"=w84, "bound_y"=w83) -> ("start_point_x"=w183:dbl, "start_point_y"=w181:dbl, "end_point_x"=w67:dbl, "end_point_y"=w66:dbl, "a"=w163:dbl, "b"=w161:dbl, "c"=w160:dbl, "curve_max_x"=→"curve_max_x":dbl, "curve_max_y"=→"curve_max_y":dbl, "curve_min_x"=→"curve_min_x":dbl, "curve_min_y"=→"curve_min_y":dbl)  [unwired: 1 in, 1 out]
        "a" <- w163
        "b" <- w161
        "c" <- w160
        "relative_end_point_x" <- w67
        "relative_end_point_y" <- w66
        "relative_end_point_x" <- w67
        "relative_end_point_y" <- w66
        n58 = Subtract(x=w35, y=w67) -> (x-y=w65:dbl)
        "error_end_point_x" <- w65
        n59 = Subtract(x=w34, y=w66) -> (x-y=w64:dbl)
        "error_end_point_y" <- w64
        n60 = Build Array(w65, w64) -> (w41:dbl[])
        "error  e(t)" <- w41
        n61 = To Double Precision Float "转换为双精度浮点数"(number=w41) -> (double precision float=w63:dbl[])
        n62 = Subtract(x=w41, y=w62) -> (x-y=w43:dbl[])
        n63 = Divide(x=w43, y="T") -> (x/y=w39:dbl[])
        n64 = Multiply(x="Kp: Proportional", y=w63) -> (x*y=w59:dbl[])
        "Kp part" <- w59
        n65 = Multiply(x="Ki: Intergrate", y=w41) -> (x*y=w42:dbl[])
        n66 = Multiply(x="Kp: Proportional", y=w39) -> (x*y=w38:dbl[])
        n67 = Multiply(x="Kd: Derivative", y=w39) -> (x*y=w57:dbl[])
        "Kd part" <- w57
        "Ki part" <- w57
        n68 = Add(x=w42, y=w44) -> (x+y=w37:dbl[])
        n69 = Add(x=w38, y=w37) -> (x+y=w36:dbl[])
        n70 = Add(x=w59, y=w36) -> (x+y=w58:dbl[])
        n71 = Add(x=w58, y=w57) -> (x+y=w45:dbl[])
        "u(t)" <- w45
        n72 = Index Array(array=w45, index=1 ("索引")) -> (element=w47:dbl)
        n73 = Index Array(array=w45, index=0 ("索引")) -> (element=w49:dbl)
        n74 = Add(x=w53, y=w49) -> (x+y=w52:dbl)
        n75 = Add(x=w52, y=w47) -> (x+y=w51:dbl)
        "magnet_input_dr" <- w51
        n76 = Add(x=w50, y=w49) -> (x+y=w48:dbl)
        n77 = Add(x=w48, y=w47) -> (x+y=w46:dbl)
        "magnet_input_pr" <- w46
        n78 = case shown="\"Rotating Field\", 默认" "Parameter Settings" {
          tunnel: w228 -> [w242 w257 w272 w291 w310 w324 w342 w357]
          tunnel: w227 -> [w239 w256 w271 w290 w308 w323 w340 w356]
          tunnel: [w241 w255 w269 w289 w309 w322 w341 w355] -> w226
          tunnel: [w240 w254 w270 w288 w307 w321 w339 w354] -> w225
          tunnel: [w235 w248 w263 w284 w301 w316 w337 w349] -> w224
          tunnel: "Pause" -> [w233 w246 w261 w283 w300 w315 w332 w347]
          tunnel: [_ _ _ w280 _ _ _ _] -> w151
          tunnel: [_ _ _ w281 _ _ _ _] -> w149
          tunnel: w54 -> [_ _ _ w279 _ _ _ _]
          tunnel: [_ _ _ w278 _ _ _ _] -> w81
          tunnel: w51 -> [_ _ _ w277 _ _ _ _]
          tunnel: w46 -> [_ _ _ w276 _ _ _ _]
          frame "Gradient Field " {
            n79 = case shown="假" w233 {
              tunnel: ["Ag" 0.0] -> w234
              frame False {
              }
              frame True {
              }
            }
            n80 = Build Array(1.0, w234, "pg", "dg", "fg") -> (w235:dbl[])
            n81 = shared-variable-write(w242, w239, w235, 1000 ("timeout ms (-1)")) -> (w241:refnum<k21>, w240:errorcluster)  [unwired: 1 out]
          }
          frame "Oscillating Field" {
            n82 = case shown="假" w246 {
              tunnel: ["AoOF" 0.0] -> w247
              frame False {
              }
              frame True {
              }
            }
            n83 = Build Array(2.0, w247, "oo", "fo", "po", "do") -> (w248:dbl[])
            n84 = shared-variable-write(w257, w256, w248, 1000 ("timeout ms (-1)")) -> (w255:refnum<k21>, w254:errorcluster)  [unwired: 1 out]
          }
          frame "Conical Field" {
            # "FG"
            n85 = case shown="假" w261 {
              tunnel: ["Ac" 0.0] -> w262
              frame False {
              }
              frame True {
              }
            }
            n86 = Build Array(3.0, w262, "wc", "pc", "dc", "cc") -> (w263:dbl[])
            n87 = shared-variable-write(w272, w271, w263, 1000 ("timeout ms (-1)")) -> (w269:refnum<k21>, w270:errorcluster)  [unwired: 1 out]
          }
          frame "Rotating Field", Default {
            n88 = case shown="假" w283 {
              tunnel: ["Ar" 0.0] -> w280
              frame False {
              }
              frame True {
              }
            }
            n89 = case shown="真" "磁场变换" {
              tunnel: [sgl 0.0 ("pr") w295] -> w286
              tunnel: [sgl 0.0 ("dr") w296] -> w281
              tunnel: w279 -> [_ w297]
              tunnel: [_ w295] -> w278
              tunnel: w277 -> [_ w296]
              tunnel: w276 -> [_ w295]
              frame False {
              }
              frame True {
                n90 = formula code="int p;\n    int q;\n    q = t/50 ;  \n    p = q%36; //用来构造循环\n    dr = -180 + (p*10);\n\n    int p2;\n    int q2;\n    q2 = q/(72);\n    p2 = q2%36; //用来构造循环\n    pr =  -40 + p2*10;"("t"=w297) -> ()  [unwired: 2 out]
                "dr" <- w296
                "pr" <- w295
              }
            }
            n91 = Build Array(4.0, w280, "wr", w286, w281) -> (w284:dbl[])
            n92 = shared-variable-write "向流中写入单个元素"(w291, w290, w284, 1000 ("timeout ms (-1)")) -> (w289:refnum<k21>, w288:errorcluster)  [unwired: 1 out]
          }
          frame "Disassembly" {
            n93 = case shown="假" w300 {
              tunnel: ["Dis strength(mT)" 0.0] -> w305
              frame False {
              }
              frame True {
              }
            }
            n94 = Build Array(5.0, w305, "Dis tumbling frequency (Hz)", "Dis phase frequency (Hz)", "Dis phase step") -> (w301:dbl[])
            n95 = shared-variable-write(w310, w308, w301, 1000 ("timeout ms (-1)")) -> (w309:refnum<k21>, w307:errorcluster)  [unwired: 1 out]
          }
          frame "Swarm" {
            n96 = case shown="假" w315 {
              tunnel: ["Swa strength (mT)" 0.0] -> w314
              frame False {
              }
              frame True {
              }
            }
            n97 = Build Array(6.0, w314, "Swa frequency (Hz)", "Swa pitch angle (deg)", "Swa direction angle (deg)", "Swa ratio") -> (w316:dbl[])
            n98 = shared-variable-write(w324, w323, w316, 1000 ("timeout ms (-1)")) -> (w322:refnum<k21>, w321:errorcluster)  [unwired: 1 out]
          }
          frame "Ribbon Oscillating Field" {
            n99 = case shown="假" w332 {
              tunnel: ["Strength (mT)" 0.0] -> w331
              frame False {
              }
              frame True {
              }
            }
            n100 = Build Array(7.0, w331, "Frequency (Hz)", "Ratio (A/C)", "Direction Angle (deg)", "Pitch Angle (rotating around Origin, deg)", "Pitch Angle (rotating around Constant, deg)") -> (w337:dbl[])
            n101 = shared-variable-write(w342, w340, w337, 1000 ("timeout ms (-1)")) -> (w341:refnum<k21>, w339:errorcluster)  [unwired: 1 out]
          }
          frame "Elliptical Field" {
            n102 = case shown="假" w347 {
              tunnel: ["Ar 2" 0.0] -> w348
              frame False {
              }
              frame True {
              }
            }
            n103 = Build Array(8.0, w348, "wr  2", "pr  2", "dr  2", "ratio", "p_x") -> (w349:dbl[])
            n104 = shared-variable-write(w357, w356, w349, 1000 ("timeout ms (-1)")) -> (w355:refnum<k21>, w354:errorcluster)  [unwired: 1 out]
          }
        }
        "Array" <- w224
        "场强" <- w151
        "dr" <- w149
        n105 = Build Array (concatenate)(w148, w149) -> (w145:dbl[])
        "direction angle" <- w145
        n106 = Build Array (concatenate)(w80, w81) -> (w79:dbl[])
        n107 = Build Array (concatenate)(w150, w151) -> (w146:dbl[])
        "strength" <- w146
        n108 = Or(x=w225, y="Stop") -> (x .or. y?=w221:bool)
        n109 = Add(x=w84, y=w183) -> (x+y=w157:dbl)
        "start_x" <- w157
        n110 = Add(x=w83, y=w181) -> (x+y=w155:dbl)
        "start_y" <- w155
        n111 = Add(x=w84, y=w67) -> (x+y=w153:dbl)
        "end_x" <- w153
        n112 = Add(x=w83, y=w66) -> (x+y=w152:dbl)
        "end_y" <- w152
        n113 = Bundle(w153, w152) -> (w169:cluster{dbl, dbl})  [unwired: 1 in]
        n114 = Bundle(w165, w155) -> (w168:cluster{i32, dbl})  [unwired: 1 in]
        n115 = Build Array(w169, w168) -> (w167:cluster{dbl, dbl}[])
        n116 = Bundle(w153, w152) -> (w69:cluster{dbl, dbl})  [unwired: 1 in]
        n117 = Build Array (concatenate)(w159, w160) -> (w143:dbl[])
        "c" <- w143
        n118 = Bundle "捆绑"(w157, w155) -> (w170:cluster{dbl, dbl})  [unwired: 1 in]
        n119 = Build Array (concatenate)(w162, w161) -> (w139:dbl[])
        "b" <- w139
        n120 = Build Array (concatenate)(w164, w163) -> (w144:dbl[])
        "a\na" <- w144
        n121 = Build Array (concatenate)(w177, w69) -> (w70:cluster{"X":dbl, "Y":dbl}[])
        n122 = Build Array (concatenate)(w74, w69) -> (w68:cluster{dbl, dbl}[])
        n123 = call "IMAQ Get Angles"("Vertex"=w170, "Points"=w167, "Use Vertex (No)"=TRUE) -> ("Angles (deg)"=→"Angles (deg)":sgl[])  [unwired: 2 in, 2 out]
        n124 = Build Array (concatenate)(w156, w157) -> (w142:dbl[])
        "start_point_x" <- w142
        n125 = Build Array (concatenate)(w154, w155) -> (w141:dbl[])
        "start_point_y" <- w141
        n126 = Build Array (concatenate)(w123, w152) -> (w131:dbl[])
        "end_point_y" <- w131
        n127 = Build Array (concatenate) "创建数组"(w127, w153) -> (w135:dbl[])
        "end_point_x" <- w135
        n128 = call "IMAQ Overlay Multiple Lines 2"("Image"=w71, "Drawing Mode (Frame)"=w75, "Color"=u32 12255487, "Width"=u32 5) -> ("Image Out"=→"仅尖端轨迹":T1)  [unwired: 10 in, 1 out]
        n129 = case shown="假" "打开仅尖端轨迹" {
          tunnel: [_ w230] -> w73
          tunnel: w68 -> [_ w230]
          frame False {
          }
          frame True {
          }
        }
        n130 = case shown="真" "打开轨迹" {
          tunnel: [_ w231] -> w172
          tunnel: w70 -> [_ w231]
          frame False {
          }
          frame True {
          }
        }
        n131 = Array Size(array=w135) -> (size(s)=w137:i32)
        n132 = call "IMAQ Overlay Multiple Lines 2"("Image"=w71, "Line End Points"=w70, "Drawing Mode (Frame)"=w82, "Color"=u32 3071, "Width"=u32 5) -> ("Image Out"=→"中心轨迹和尖端轨迹":T1)  [unwired: 9 in, 1 out]
        n133 = Array Size(array=w131) -> (size(s)=w133:i32)
        n134 = Subtract(x=w137, y=1) -> (x-y=w136:i32)
        n135 = Subtract(x=w133, y=1) -> (x-y=w132:i32)
        n136 = Index Array "索引数组"(array=w135, index=w136) -> (element=w122:dbl)
        "now_end_point_x" <- w122
        n137 = Subtract "delta_x"(x=w122, y=w121) -> (x-y=w93:dbl)
        "delta_x" <- w93
        n138 = Build Array (concatenate) "delta_x"(w114, w93) -> (w112:dbl[])
        n139 = Square(x=w93) -> (x^2=w118:dbl)
        n140 = Index Array "索引数组"(array=w131, index=w132) -> (element=w119:dbl)
        "now_end_point_y" <- w119
        n141 = Subtract "delta_y"(x=w119, y=w120) -> (x-y=w92:dbl)
        "delta_y" <- w92
        n142 = Build Array (concatenate) "delta_y"(w113, w92) -> (w111:dbl[])
        n143 = Square(x=w92) -> (x^2=w117:dbl)
        n144 = Add(x=w118, y=w117) -> (x+y=w116:dbl)
        n145 = Square Root(x=w116) -> (sqrt(x)=w115:dbl)
        "delta_distance" <- w115
        n146 = Divide(x=w93, y=w92) -> (x/y=w91:dbl)
        "tan(v)" <- w91
        n147 = Divide(x=w115, y=w97) -> (x/y=w96:dbl)
        "delta_velocity" <- w96
        n148 = Build Array (concatenate)(w90, w91) -> (w89:dbl[])
        n149 = Build Array (concatenate) "delta_velocity"(w95, w96) -> (w94:dbl[])
        n150 = Build Array(w147, w146, w145, w144, w139, w143, w142, w141, w135, w131, w112, w111, w98, w94, w89, w79) -> (→"all parameters":dbl[][])
        "Numeric 5" <- w54
        "T" <- w54
        "T" <- w54
        "prev_end_point_x" <- w127
        "prev_end_point_y" <- w123
        "prev time" <- w106
        "e(t-1)" <- w62
      }
    }
    frame #3 {
      # "4. The error -314220 indicates that the other endpoint has been destroyed. The VI ignores this error."
      # "3. Destroy the stream endpoint when you click Stop or when an error occurs."
      # "Close"
      n151 = Flush Stream(8:w367, 11:w370) -> (0:w368:errorcluster, 3:w369:refnum<k21>)  [unwired: 2 in, 1 out]
      n152 = Destroy Stream Endpoint(8:w368, 11:w369) -> (0:w362:errorcluster)
      n153 = Unbundle By Name(w362) -> ("code"=w366:i32)
      n154 = xnode "Error Ring"() -> ("错误输出"=w363:errorcluster)
      n155 = Not Equal?(x=w366, y=-314220) -> (x != y?=w364:bool)
      n156 = Select(t=w362, s=w364, f=w363) -> (s? t:f=→"error out":errorcluster)
    }
  }
